vi "Find Item in Library.vi"(7 "Item Type":string, 8 "error in (no error)":errorcluster, 10 "Item Name":string, 11 "Library item in":refnum<vi>) -> (0 "error out":errorcluster, 1 "Found?":bool, 2 "Project Item (Library Item)":refnum<vi>, 3 "Library item out":refnum<vi>)   [LabVIEW 2019, in "gRPC Scripting Tools.lvlib"]
uses:
  gRPC Scripting Tools.lvlib
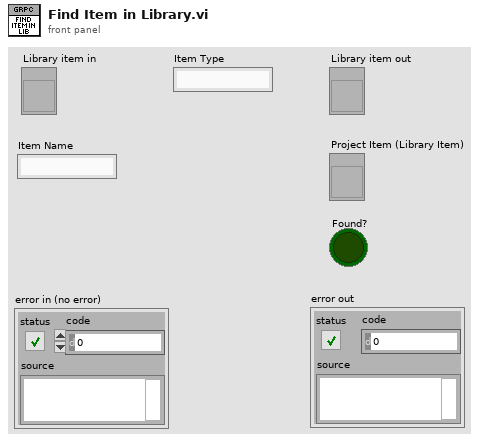
[diagram p1: front panel]
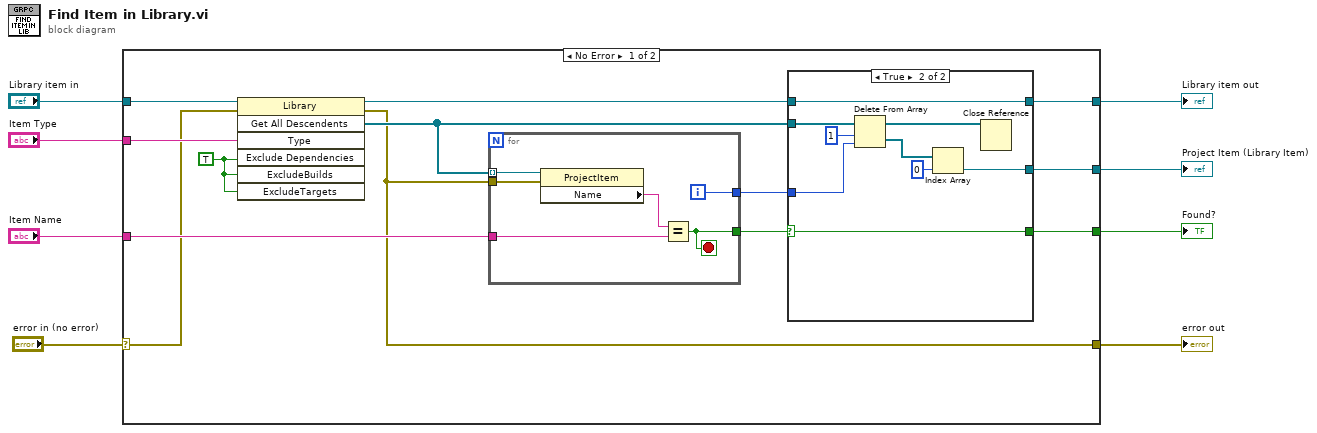
[diagram p0: block diagram]
diagram:
  n1 = case shown="No Error" "error in (no error)" {
    selector: "error in (no error)" -> [w15 w38]
    tunnel: "Item Name" -> [w21 _]
    tunnel: "Item Type" -> [w17 _]
    tunnel: "Library item in" -> [w16 w39]
    tunnel: [w10 w39] -> w2
    tunnel: [w12 _] -> w4
    tunnel: [w14 _] -> w3
    tunnel: [w9 w38] -> w1
    frame No Error {
      w18 = TRUE ("ExcludeDependencies")
      n2 = invoke class="Library" method="Get All Descendents"(reference=w16, error in=w15, "Type"=w17, "Exclude Dependencies"=w18, "ExcludeBuilds"=w18, "ExcludeTargets"=w18) -> (reference out=w11:refnum<vi>, error out=w9:errorcluster, "All Descendents"=w19:refnum<vi>[])  [unwired: 1 in, 4 out]
      n3 = for {
        tunnel: w19 -> [w37] mode=indexing
        tunnel: [w35] -> w20
        tunnel: [w34] -> w13
        tunnel: w21 -> [w33]
        tunnel: w9 -> [w32]
        i -> [w35]
        stop <- w34 stop-if-true
        n4 = property class="ProjectItem"(reference=w37, error in=w32) -> ("Name"=w36:string)  [unwired: 2 out]
        n5 = Equal?(x=w36, y=w33) -> (x = y?=w34:bool)
      }
      n6 = case shown="True" w13 {
        selector: w13 -> [_ w24]
        tunnel: w20 -> [_ w29]
        tunnel: w19 -> [_ w28]
        tunnel: [_ w25] -> w14
        tunnel: [_ w24] -> w12
        tunnel: w11 -> [w22 w23]
        tunnel: [w22 w23] -> w10
        frame False {
        }
        frame True {
          n7 = Delete From Array(array=w28, length=1, index=w29) -> (deleted portion=w27:refnum<vi>[], array with subset deleted=w31:refnum<vi>[])
          n8 = Index Array(array=w27, index=0) -> (element=w25:refnum<vi>)
          n9 = Close Reference(reference=w31) -> ()  [unwired: 1 in, 1 out]
        }
      }
    }
    frame Error {
    }
  }
  "Project Item (Library Item)" <- w3
  "Found?" <- w4
  "Library item out" <- w2
  "error out" <- w1
